vi "Sort scaling sensors.vi"(0 "Channels in":T2={"DAQ Settings"={"Trigger Type"=enum."Manual", "Trigger Samples"=0, "Pretrigger Samples"=0, "Trigger Interval"=0.0, "Time Units"=FALSE, "Auto Save"=FALSE, "Sample Rate"=7.0, "Select Analog"=FALSE, "Trigger Value"=0.0, "Trigger Stop Method"=enum."Use Samples Value to Stop Trigger", "Rate Sec/Min"=FALSE, "Save Mode"=enum."Single File", "File Size Limit"=0.0, "Log File Type"=enum."Basic", "Trigger Data Index"=0, "Log Rate"=7.0, "Rate Sec/Min (Log)"=FALSE, "Sample Rate (S/s)"=0.0, "Log Rate (S/s)"=0.0}, "Channels"=[], "Header"={"CA Number"="", "Test Name"="", "Serial Number"="", "Technician"=""}, "Graph Settings"={"Graph Labels"=[], [], [], [], [], [], [], [], [], [], [], [], [], "Graph Toggles"=[], "Axis Toggles"=[], "Graph Range"=enum."1"}, "Test Limits"=[], "All Type Info"=[], "Save Mode"=enum."Single File", "Data Base Path"=path ""} {"DAQ Settings"."Trigger Interval" min=0.0; "DAQ Settings"."Pretrigger Samples" min=0; "DAQ Settings"."Trigger Samples" min=0}, 1 "Sensors (scale)":T1(array[cluster]) {"Max Error % of Reading" format="%.2f"; "Max Stability Error" format="%.2f"; "Max Mean Squared Error" format="%.2f"; "Max Error % of Full Scale" format="%.2f"; "Coefficients" format="%.2f"; "Voltage List" format="%.2f"; "EGU List" format="%.2f"; "EGU Range"."Low Limit" format="%.2f"; "EGU Range"."High Limit" format="%.2f"; "Voltage Range"."Low Limit" format="%.2f"; "Voltage Range"."High Limit" format="%.2f"; "Last Cal Info"."Last Calibration Date" format="%.2f"}) -> (14 "Sensor (scaling) out":T1(array[cluster]))   [LabVIEW 2023]
uses:
  Type Defs and Controls/Sensor Config.ctl
  Type Defs and Controls/DAQ Settings.ctl
  Type Defs and Controls/Trigger Stop Method.ctl
  Type Defs and Controls/Log File Type.ctl
  Type Defs and Controls/Channel Config.ctl
  Type Defs and Controls/Header.ctl
  Type Defs and Controls/Graph Settings Type Def.ctl
  Type Defs and Controls/Test Limits.ctl
  Type Defs and Controls/All Part Info.ctl
  Type Defs and Controls/Part Info.ctl
panel:
  # "EGU"
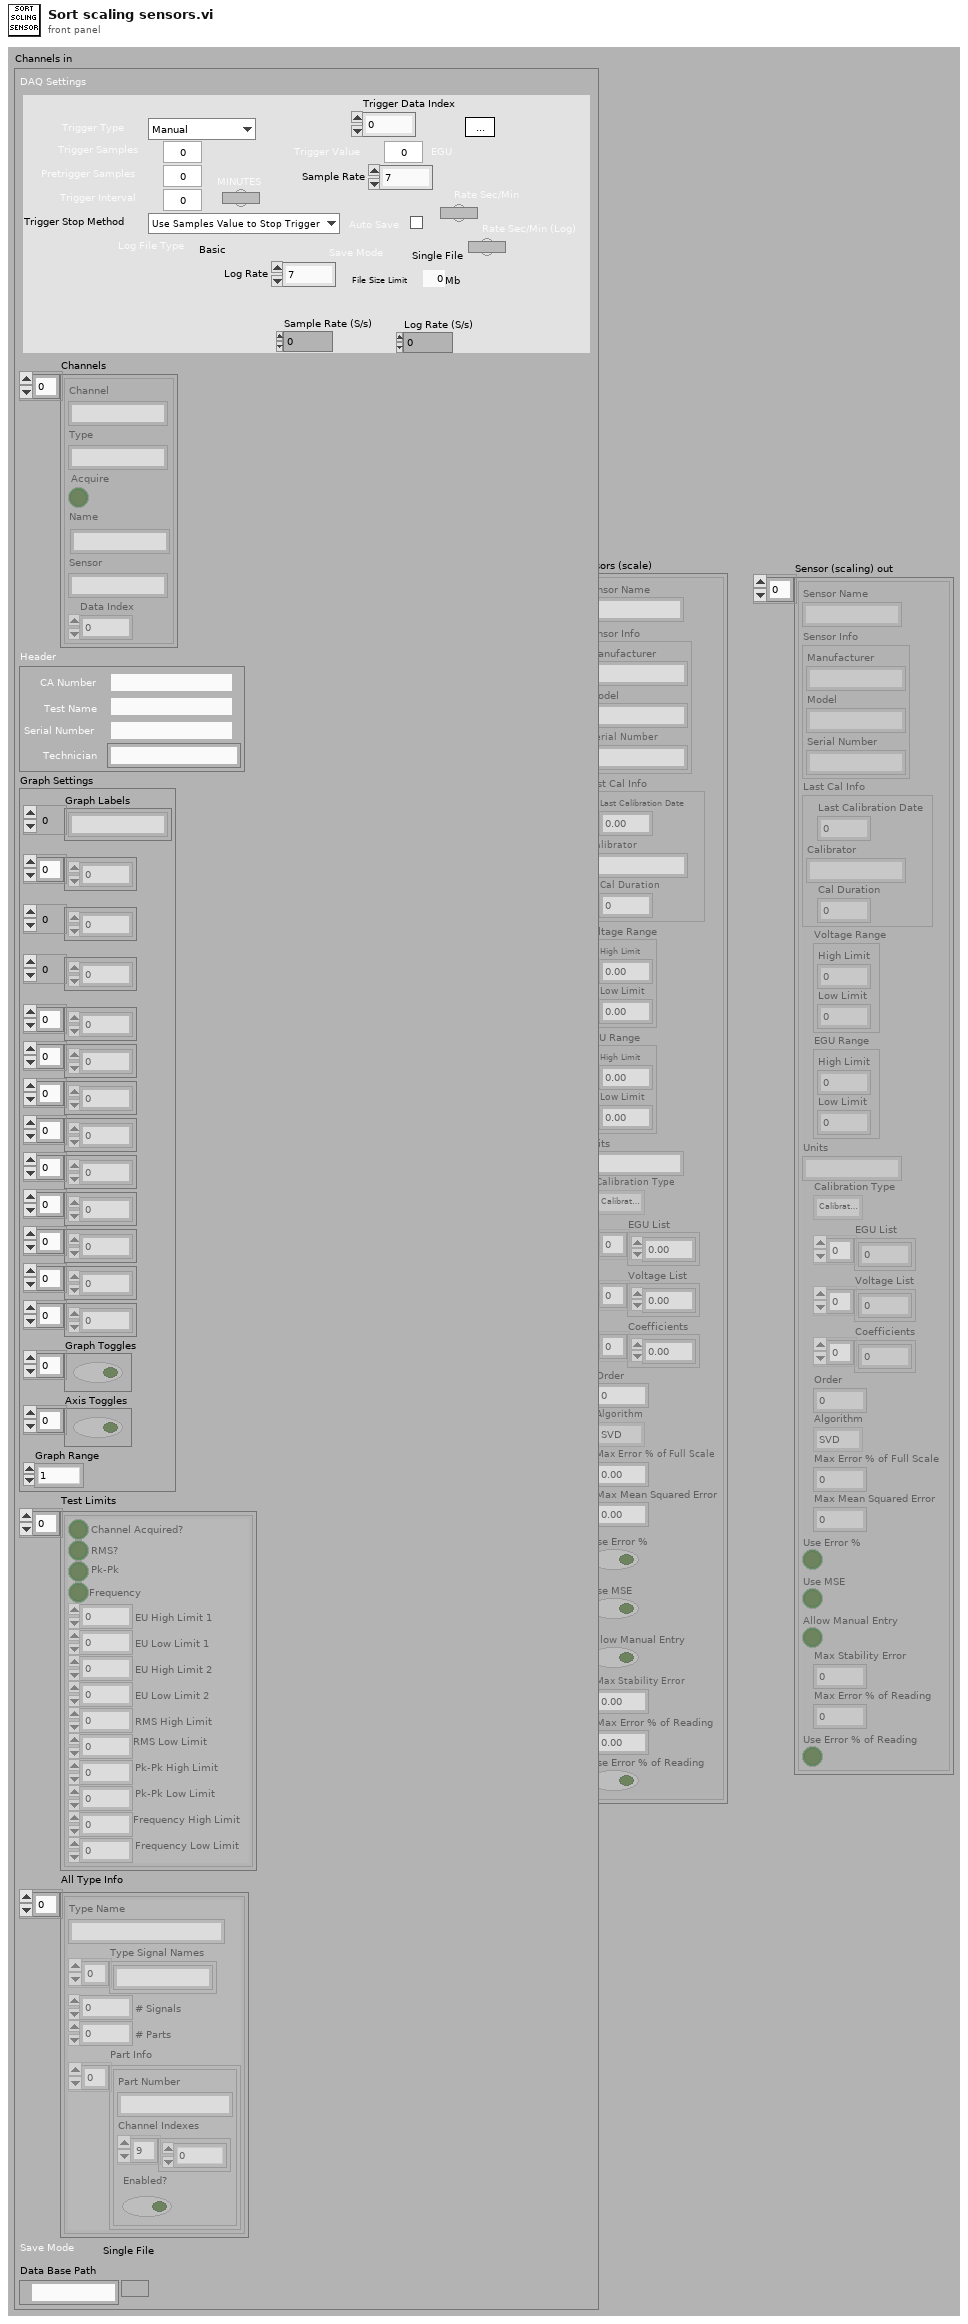
[diagram p1: front panel]
types:
  T1 = cluster{"Sensor Name":string, "Sensor Info":cluster{"Manufacturer":string, "Model":string, "Serial Number":string}, "Last Cal Info":cluster{"Last Calibration Date":dbl, "Calibrator":string, "Cal Duration":i32}, "Voltage Range":cluster{"High Limit":dbl, "Low Limit":dbl}, "EGU Range":cluster{"High Limit":dbl, "Low Limit":dbl}, "Units":string, "Calibration Type":enum16{"Calibrate Analog", "Compare Analog Calibration"}, "EGU List":dbl[], "Voltage List":dbl[], "Coefficients":dbl[], "Order":i32, "Algorithm":enum32{"SVD", "Givens", "Givens2", "Householder", "LU Decomposition", "Cholesky"}, "Max Error % of Full Scale":dbl, "Max Mean Squared Error":dbl, "Use Error %":bool, "Use MSE":bool, "Allow Manual Entry":bool, "Max Stability Error":dbl, "Max Error % of Reading":dbl, "Use Error % of Reading":bool}[]
  T2 = typedef "Sensor Config.ctl" = cluster{"DAQ Settings":T3, "Channels":T6[], "Header":T7, "Graph Settings":T8, "Test Limits":T9[], "All Type Info":T10, "Save Mode":enum16{"Single File", "Segmented Files", "New File at Midnight"}, "Data Base Path":path}
  T3 = typedef "DAQ Settings.ctl" = cluster{"Trigger Type":enum16{"Manual", "Timed", "Analog Rising", "Analog Falling"}, "Trigger Samples":i32, "Pretrigger Samples":i32, "Trigger Interval":dbl, "Time Units":bool, "Auto Save":bool, "Sample Rate":dbl, "Select Analog":bool, "Trigger Value":dbl, "Trigger Stop Method":T4, "Rate Sec/Min":bool, "Save Mode":enum16{"Single File", "Segmented Files", "New File at Midnight"}, "File Size Limit":dbl, "Log File Type":T5, "Trigger Data Index":u32, "Log Rate":dbl, "Rate Sec/Min (Log)":bool, "Sample Rate (S/s)":dbl, "Log Rate (S/s)":dbl}
  T4 = typedef "Trigger Stop Method.ctl" = enum16{"Use Samples Value to Stop Trigger", "Use Threshold to Stop Trigger"}
  T5 = typedef "Log File Type.ctl" = enum16{"Basic", "RTS"}
  T6 = typedef "Channel Config.ctl" = cluster{"Channel":string, "Type":string, "Acquire":bool, "Name":string, "Sensor":string, "Data Index":u32}
  T7 = typedef "Header.ctl" = cluster{"CA Number":string, "Test Name":string, "Serial Number":string, "Technician":string}
  T8 = typedef "Graph Settings Type Def.ctl" = cluster{"Graph Labels":string[], u8[], i16[], u32[], u8[], u8[], u8[], u32[], u8[], u8[], u8[], dbl[], dbl[], "Graph Toggles":bool[], "Axis Toggles":bool[], "Graph Range":enum16{"1", "2", "3", "4", "5", "10", "15", "30", "60"}}
  T9 = typedef "Test Limits.ctl" = cluster{"Channel Acquired?":bool, "RMS?":bool, "Pk-Pk":bool, "Frequency":bool, "EU High Limit 1":dbl, "EU Low Limit 1":dbl, "EU High Limit 2":dbl, "EU Low Limit 2":dbl, "RMS High Limit":dbl, "RMS Low Limit":dbl, "Pk-Pk High Limit ":dbl, "Pk-Pk Low Limit":dbl, "Frequency High Limit":dbl, "Frequency Low Limit":dbl}
  T10 = typedef "All Part Info.ctl" = cluster{"Type Name":string, "Type Signal Names":string[], "# Signals":i32, "# Parts":i32, "Part Info":T11[]}[]
  T11 = typedef "Part Info.ctl" = cluster{"Part Number":string, "Channel Indexes":u16[], "Enabled?":bool}
  T12 = cluster{"Sensor Name":string, "Sensor Info":cluster{"Manufacturer":string, "Model":string, "Serial Number":string}, "Last Cal Info":cluster{"Last Calibration Date":dbl, "Calibrator":string, "Cal Duration":i32}, "Voltage Range":cluster{"High Limit":dbl, "Low Limit":dbl}, "EGU Range":cluster{"High Limit":dbl, "Low Limit":dbl}, "Units":string, "Calibration Type":enum16{"Calibrate Analog", "Compare Analog Calibration"}, "EGU List":dbl[], "Voltage List":dbl[], "Coefficients":dbl[], "Order":i32, "Algorithm":enum32{"SVD", "Givens", "Givens2", "Householder", "LU Decomposition", "Cholesky"}, "Max Error % of Full Scale":dbl, "Max Mean Squared Error":dbl, "Use Error %":bool, "Use MSE":bool, "Allow Manual Entry":bool, "Max Stability Error":dbl, "Max Error % of Reading":dbl, "Use Error % of Reading":bool}
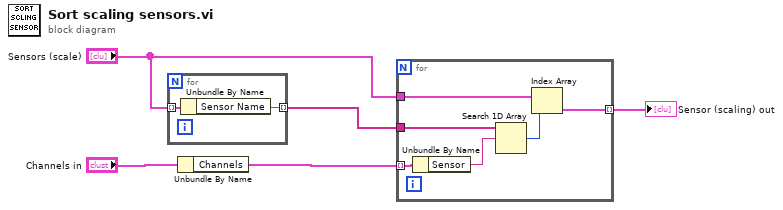
[diagram p0: block diagram]
diagram:
  n1 = for {
    tunnel: "Sensors (scale)" -> [w7] mode=indexing
    tunnel: [w6] -> w2 mode=indexing
    n2 = Unbundle By Name(w7) -> ("Sensor Name"=w6:string)
  }
  n3 = Unbundle By Name("Channels in") -> ("Channels"=w4:T6[])
  n4 = for {
    tunnel: w4 -> [w12] mode=indexing
    tunnel: w2 -> [w13]
    tunnel: "Sensors (scale)" -> [w9]
    tunnel: [w8] -> w1 mode=indexing
    n5 = Unbundle By Name(w12) -> ("Sensor"=w11:string)
    n6 = Search 1D Array(1D array=w13, element=w11) -> (index of element=w10:i32)  [unwired: 1 in]
    n7 = Index Array(array=w9, index=w10) -> (element=w8:T12)
  }
  "Sensor (scaling) out" <- w1
